vi "Read Teller.vi"(11 "Stop Msg Input in":refnum<class "Stop Msg Input.lvclass">) -> (2 "Teller":refnum<class "Teller.lvclass">)   [LabVIEW 2020, in "jettl.lvlib" / "Stop jettl Msg.lvlib" / "Stop Msg Input.lvlib" / "Stop Msg Input.lvclass"]
uses:
  Stop Msg Input.lvclass
  Teller/Teller.lvclass
  Stop Msg Input.lvclass/Stop Msg Input.ctl
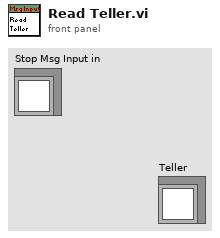
[diagram p1: front panel]
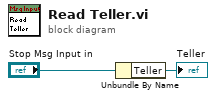
[diagram p0: block diagram]
diagram:
  n1 = Unbundle By Name("Stop Msg Input in") -> ("Teller"=→"Teller":refnum<class "Teller.lvclass">)
